vi "read_config.vi"   [LabVIEW 2017]
uses:
  <vilib>/Utility/config.llb/Read Key (String).vi
  admin_settings.vi
  <vilib>/Utility/config.llb/Read Key (Boolean).vi
  <vilib>/Utility/config.llb/Read Key (I32).vi
  <vilib>/Utility/config.llb/NI_LVConfig.lvlib
types:
  T1 = typedef "NI_LVConfig.lvlib/Config Data RefNum.ctl" = refnum<k1>
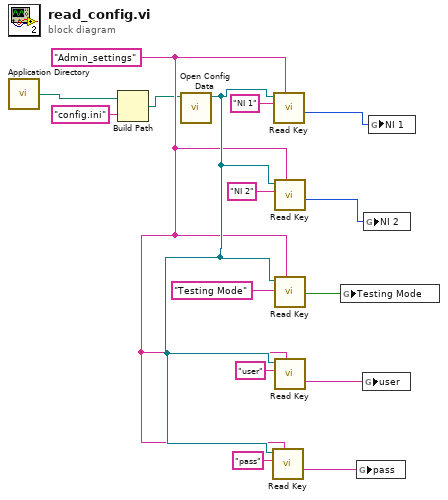
[diagram p0: block diagram]
diagram:
  w12 = "Admin_settings" ("section")
  n1 = call <vilib>:"Application Directory.vi"() -> ("Application Directory"=w4:path)
  n2 = Build Path(base path=w4, name or relative path="config.ini") -> (appended path=w5:path)
  n3 = call <vilib>:"Open Config Data.vi"("configuration file path"=w5) -> ("refnum"=w15:T1)  [unwired: 8 in, 2 out]
  n4 = call-poly <vilib>:"Read Key.vi"("section"=w12, "key"="pass", "refnum"=w15) -> ("value"=w11:string)  [unwired: 5 in, 3 out]
  n5 = call-poly <vilib>:"Read Key.vi"("section"=w12, "key"="NI 1", "refnum"=w15) -> ("value"=w3:i32)  [unwired: 5 in, 3 out]
  n6 = call-poly <vilib>:"Read Key.vi"("section"=w12, "key"="NI 2", "refnum"=w15) -> ("value"=w2:i32)  [unwired: 5 in, 3 out]
  n7 = call-poly <vilib>:"Read Key.vi"("section"=w12, "key"="Testing Mode", "refnum"=w15) -> ("value"=w1:bool)  [unwired: 5 in, 3 out]
  n8 = call-poly <vilib>:"Read Key.vi"("section"=w12, "key"="user", "refnum"=w15) -> ("value"=w10:string)  [unwired: 5 in, 3 out]
  n9 = global write "admin_settings.vi" "Testing Mode"(w1) -> ()
  n10 = global write "admin_settings.vi" "pass"(w11) -> ()
  n11 = global write "admin_settings.vi" "user"(w10) -> ()
  n12 = global write "admin_settings.vi" "NI 2"(w2) -> ()
  n13 = global write "admin_settings.vi" "NI 1"(w3) -> ()
